vi "Main2_beforerefactoring.vi"() -> ()   [LabVIEW 2021]
uses:
  Hamamatsu_class/SubRegion.ctl
  Application_class/Application.lvclass
  CetoniPump_class/CetoniPump.lvclass
  <vilib>/vision/Image Controls.llb/IMAQ Image.ctl
  Coriolis_Sim_class/Coriolis_Sim.lvclass
  C:/GIT/DensityGradientProject/CoriFlowBFS1Plus_class/CoriFlowBFS1Plus.lvclass
  CoriFlowBFS1Plus_class/CoriFlowBFS1Plus.lvclass
  <vilib>/Utility/error.llb/Error Cluster From Error Code.vi
  <vilib>/ErrorRing/Error Ring.xnode
  AD2_SDK_class/AD2_SDK.lvclass
  Hamamatsu_class/Hamamatsu.lvclass
panel:
  out "Density_g_L":sgl
  out "Temperature(C)":sgl
  out "FLow(ul/min)":sgl
  out "Status":string
  out "Array":T1(array[cluster])
  out "error out":errorcluster
  in  "Tab Control":T2(tab)
  in  "Read Continous":bool
  in  "Go to Level":bool
  in  "Device Configuration Path":string="C:\\Users\\Public\\Documents\\QmixElements\\Projects\\default_project\\Configurations\\double"
  in  "Go to Level":T3
  in  "index":i32
  in  "ReferenceMove":bool
  in  "ReadStatus":bool
  in  "ConfigureSyringe":bool
  in  "SyringeSettings":T4={"index"=0, "SyringeSettings"={"Maximum Piston Stroke (mm)"=100.0, "Inner Diameter (mm)"=12.0}}
  in  "Syringe (only for syringe helper)":T5(ring)=enum."BD 5ml"
  out "Syringe Helper":T6={"Maximum Piston Stroke (mm)"=48.147993421803335, "Inner Diameter (mm)"=12.06}
  in  "Stop ALL Pumps":bool
  in  "CetoniWaitData":T7
  in  "Cetoni Wait for Level":bool
  in  "Center ROI":bool
  in  "Configure ROI":bool
  in  "ROI":T8
  in  "StartLive":bool
  in  "Stop Live":bool
  in  "Open DIO signal helper":bool
  in  "Set Exposure Time":bool
  in  "Read Redout Time":bool
  out "ReadoutTime":dbl
  in  "Exposure (ms)":dbl=5.0 step=1.0
  in  "Start HW Timed Aquisition":bool
  in  "Triggering":T9
  in  "Read Continously?":bool
  in  "Read Coriolis":bool
  in  "Use Coriolis?":bool
  in  "Coriolis VISA resource name":refnum<visa-resource-name>
  in  "Filter(0-1)Min-Max":dbl min=0.0 max=1.0
  out "Display <Replace Me> 2":string
  in  "Exit":bool
  in  "Inject Error<Replace Me>":bool
  in  "Do Something <Replace Me>":bool
  # "DIO0 Pulses at the same time as DIO1,2 and 3 +-offset"
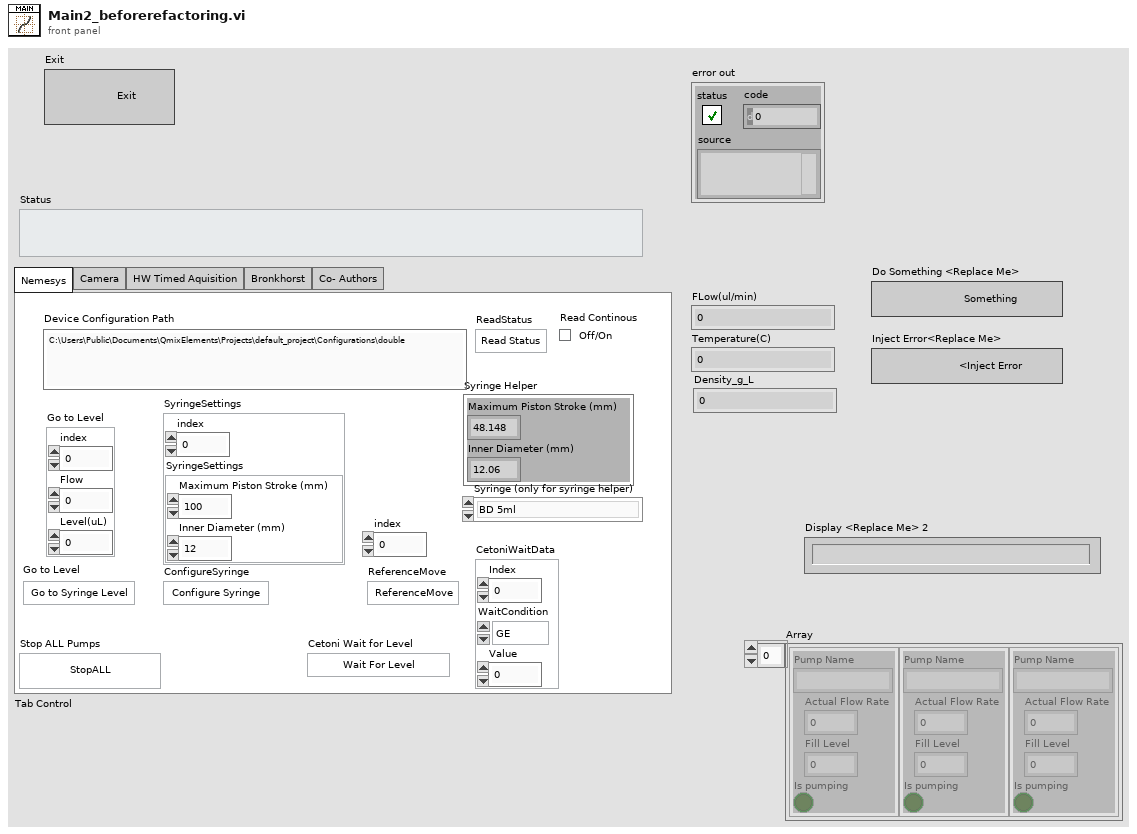
[diagram p1: front panel]
types:
  T1 = cluster{"Pump Name":string, "Actual Flow Rate":dbl, "Fill Level":dbl, "Is pumping":bool}[]
  T2 = enum32{"Nemesys", "Camera", "HW Timed Aquisition", "Bronkhorst", "Co- Authors"}
  T3 = cluster{"index":i32, "Flow":dbl, "Level(uL)":dbl}
  T4 = cluster{"index":i32, "SyringeSettings":cluster{"Maximum Piston Stroke (mm)":dbl, "Inner Diameter (mm)":dbl}}
  T5 = enum16{"BD 1ml", "BD 3ml", "BD 5ml", "BD 10ml", "BD 20ml", "BD 30ml", "BD 50ml", "HSW 1ml"}
  T6 = cluster{"Maximum Piston Stroke (mm)":dbl, "Inner Diameter (mm)":dbl}
  T7 = cluster{"Index":u8, "WaitCondition":enum16{"GE", "LE", "Stopped"}, "Value":dbl}
  T8 = typedef "Hamamatsu.lvclass/SubRegion.ctl" = cluster{"Horizontal Offset":i32, "Vertical Offset":i32, "Horizontal Size":i32, "Vertical Size":i32}
  T9 = cluster{"Pulse Length(ms)":dbl, "DIO0Offset(ms)":dbl, "DIO1 Pulse time (ms)":dbl, "DIO2 Pulse time (ms) 2":dbl, "DIO3 Pulse time (ms) 3":dbl, "EnableDIO3":bool, "EnableDIO2":bool, "EnableDIO1":bool}
  T10 = cluster{"Message":string, "Message Data":variant}
  T11 = cluster{"Fill Level":dbl, "Is pumping":bool, "Actual Flow Rate":dbl}
  T12 = typedef "LVMinMaxIncTypeDef.ctl" = cluster{"Minimum":dbl, "Maximum":dbl, "Increment":dbl}
  T13 = cluster{"H Offset":cluster{"Value":i32, "Limits":T12}, "V Offset":cluster{"Value":i32, "Limits":T12}, "H Size":cluster{"Value":i32, "Limits":T12}, "V Size":cluster{"Value":i32, "Limits":T12}}
  T14 = typedef "Hamamatsu.lvclass/SubRegionLimits.ctl" = cluster{"H Offset":cluster{"Value":i32, "Limits":T12}, "V Offset":cluster{"Value":i32, "Limits":T12}, "H Size":cluster{"Value":i32, "Limits":T12}, "V Size":cluster{"Value":i32, "Limits":T12}}
  T15 = typedef "IMAQ Image.ctl" = refnum<image>
  T16 = enum32{"Invalid", "Standard", "Closed", "Hidden", "Minimized", "Maximized"}
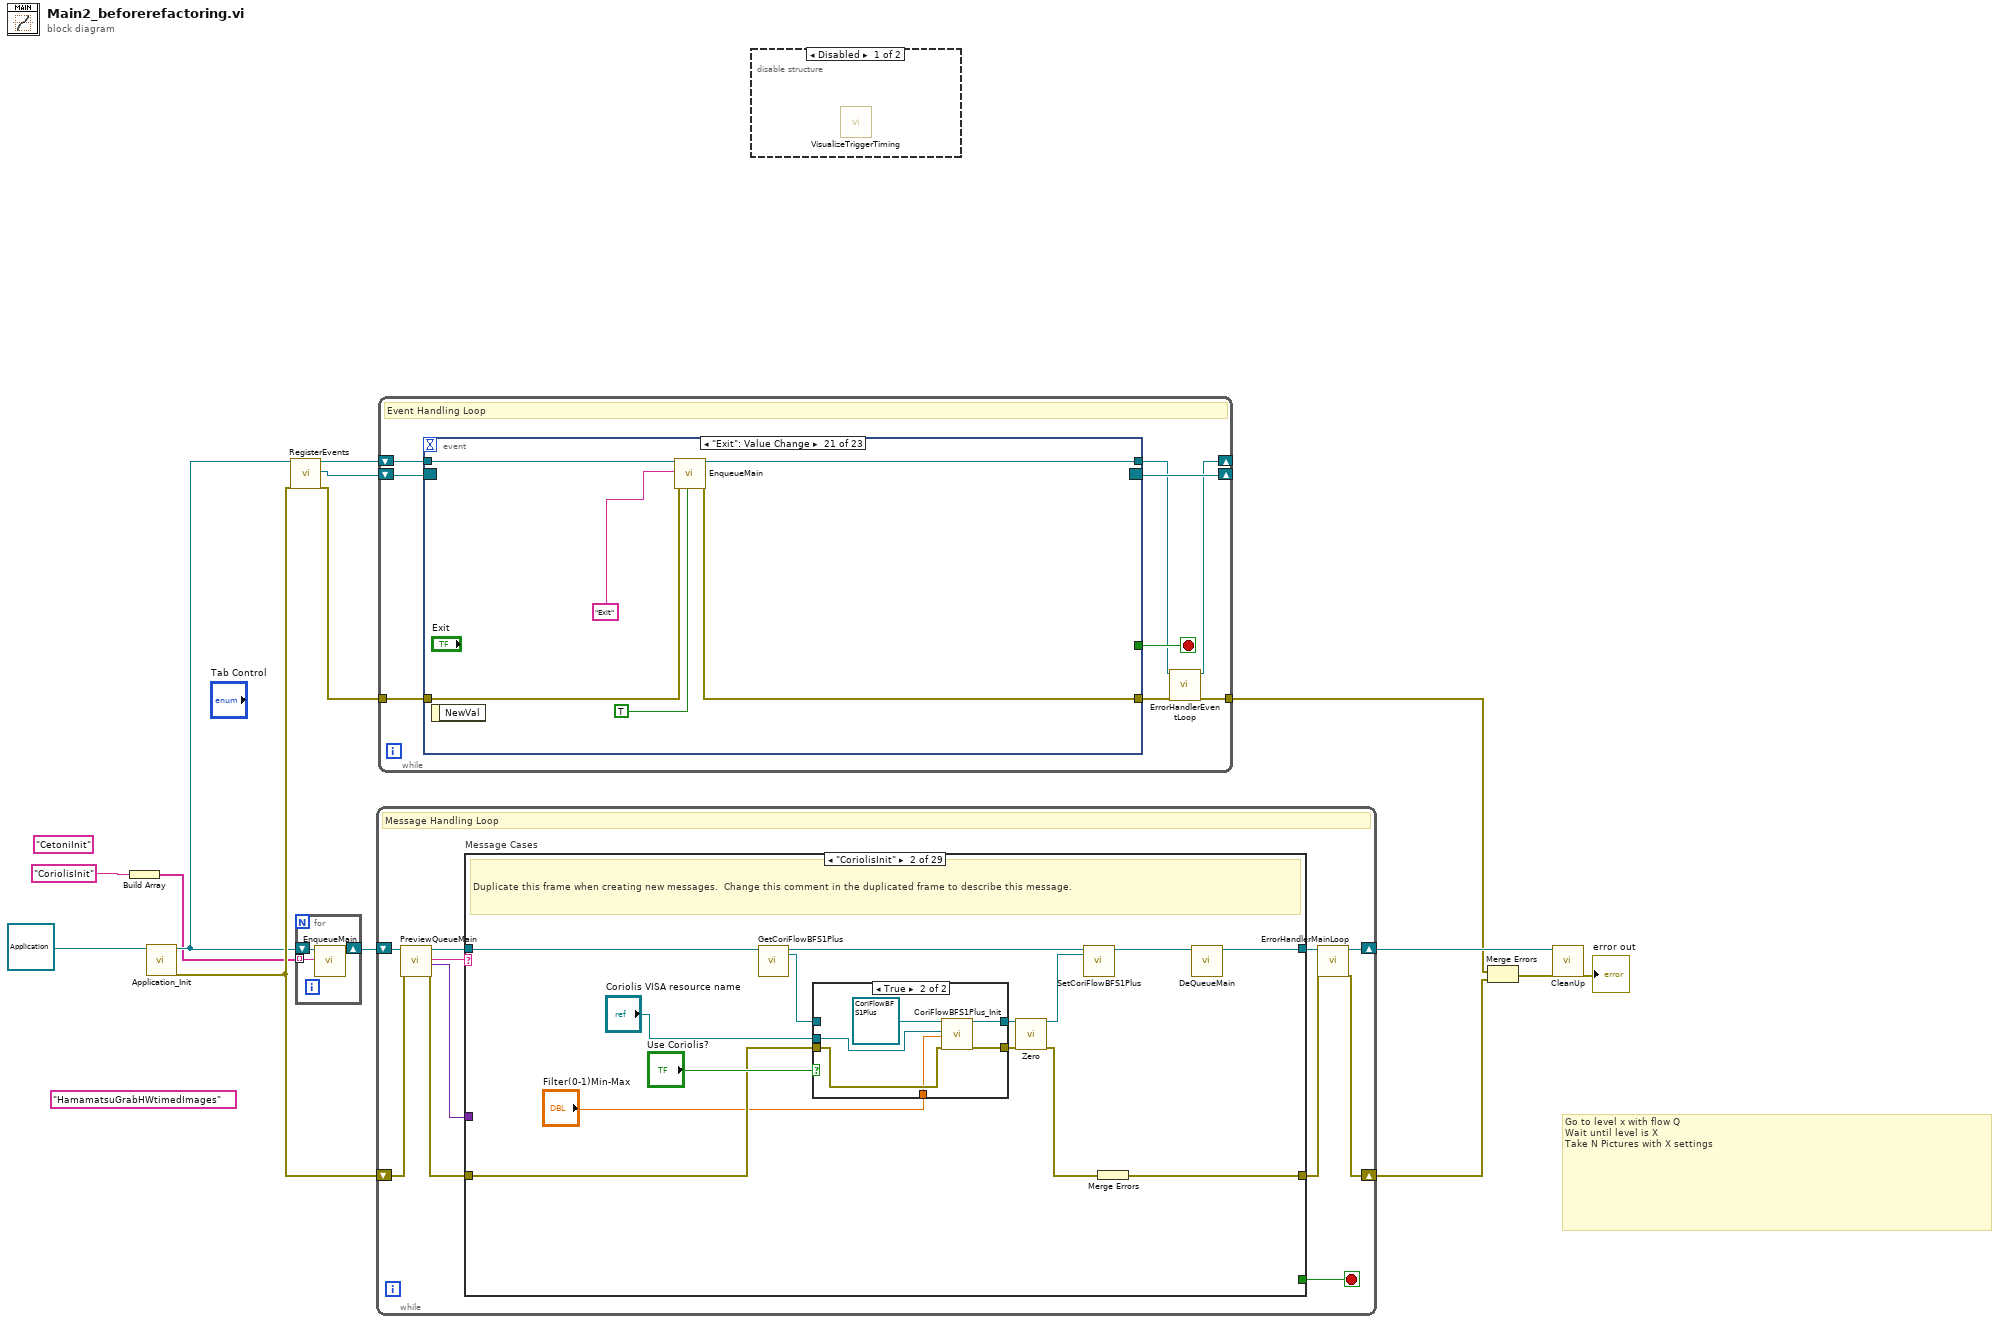
[diagram p0: block diagram]
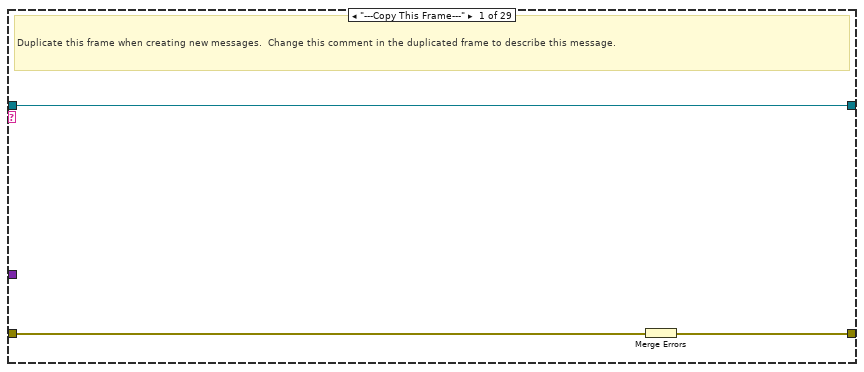
[diagram p3: hidden frame]
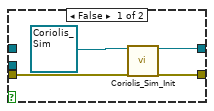
[diagram p4: hidden frame]
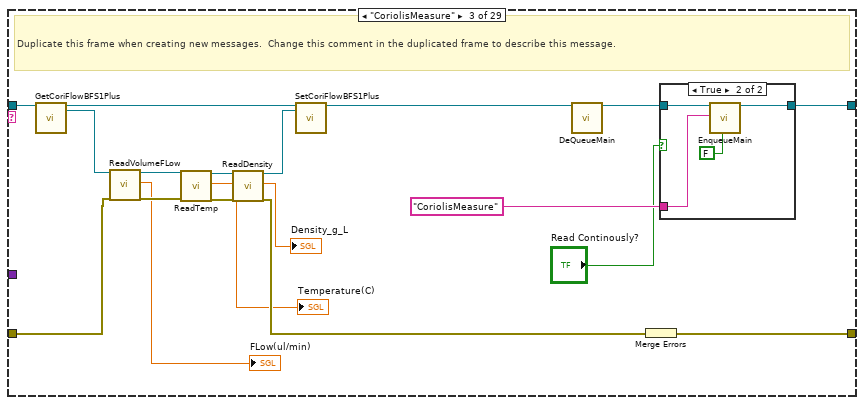
[diagram p5: hidden frame]
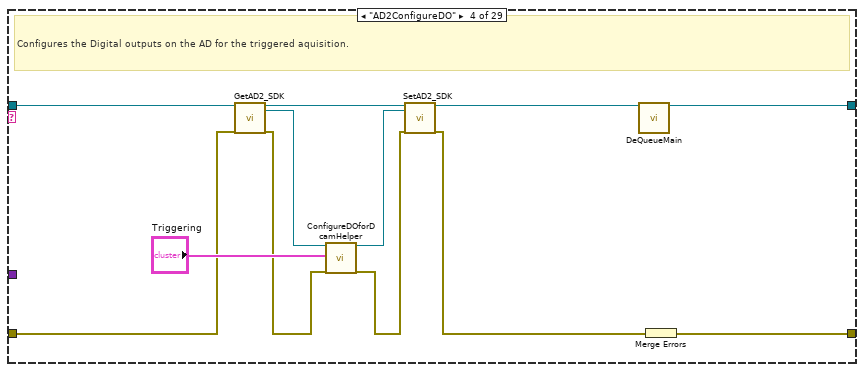
[diagram p7: hidden frame]
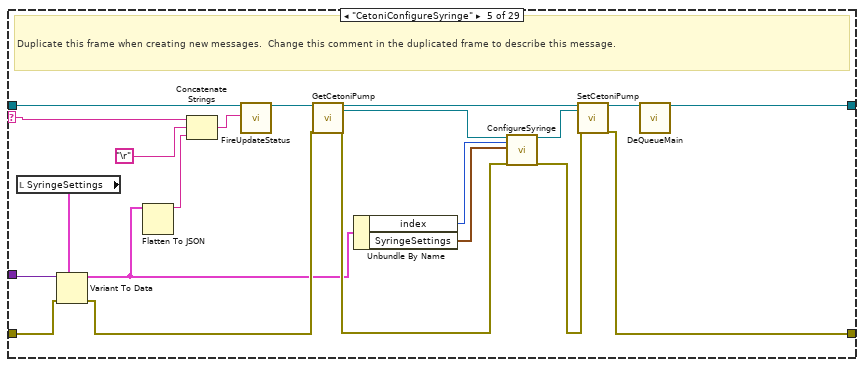
[diagram p8: hidden frame]
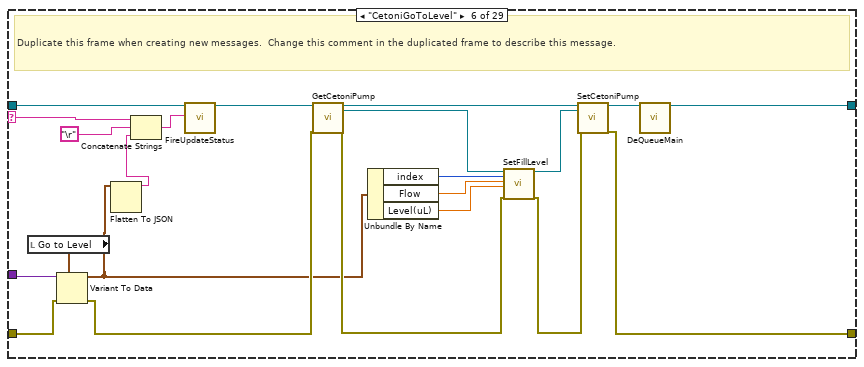
[diagram p9: hidden frame]
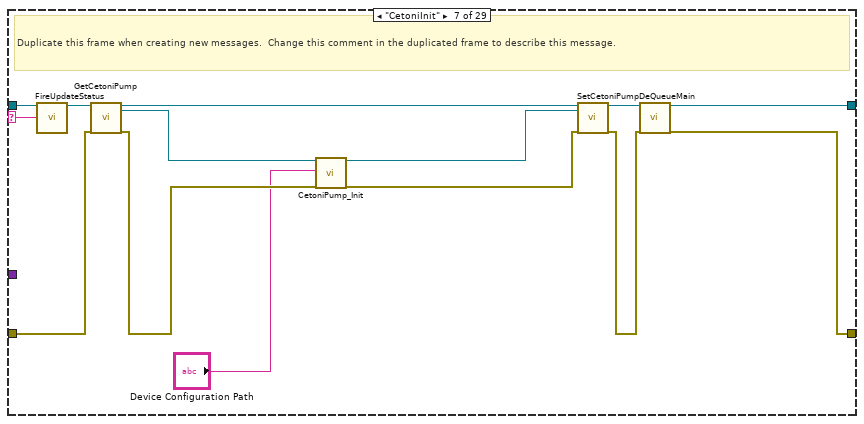
[diagram p10: hidden frame]
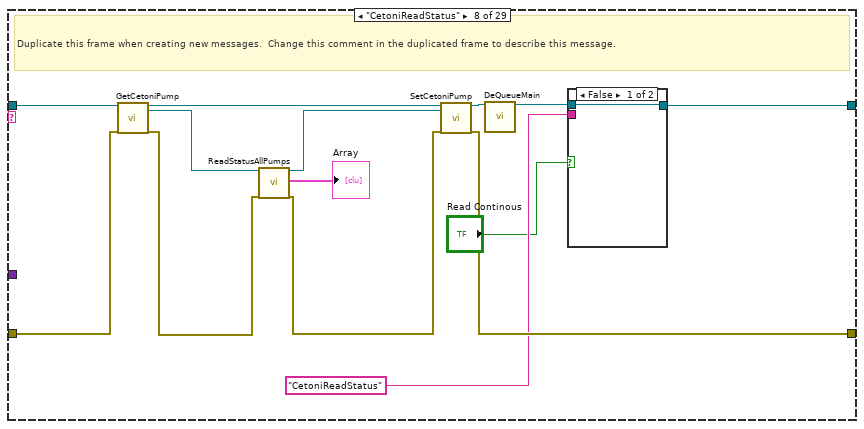
[diagram p11: hidden frame]
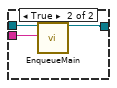
[diagram p12: hidden frame]
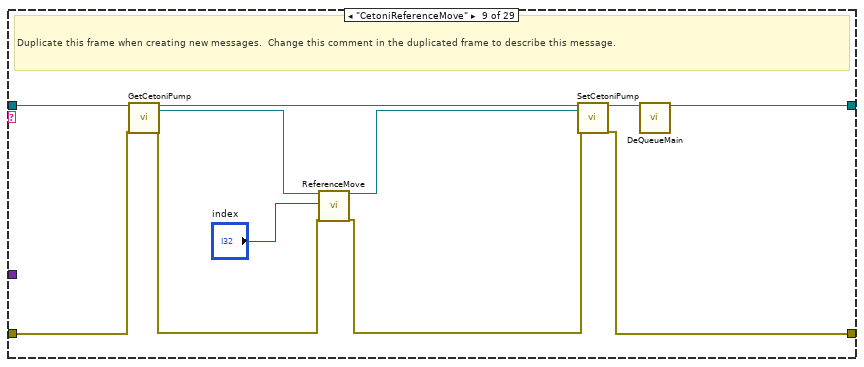
[diagram p13: hidden frame]
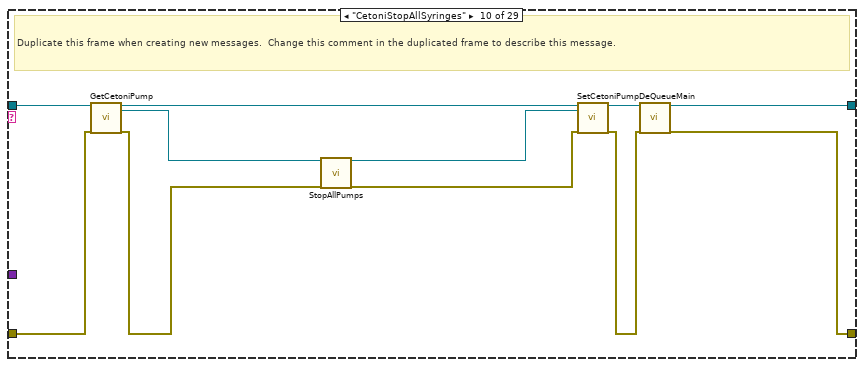
[diagram p14: hidden frame]
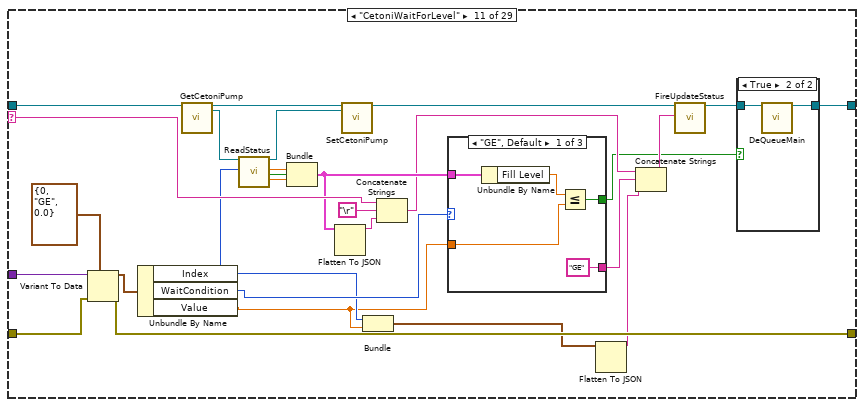
[diagram p15: hidden frame]
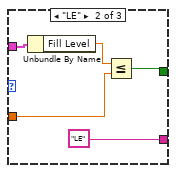
[diagram p17: hidden frame]
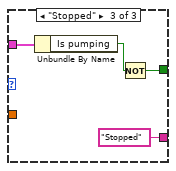
[diagram p18: hidden frame]
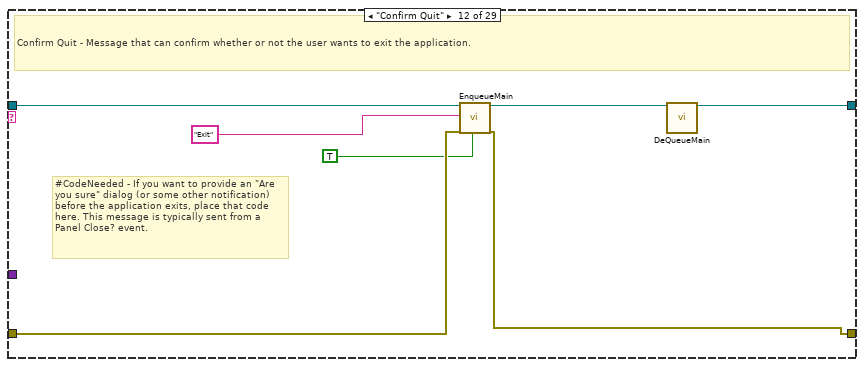
[diagram p19: hidden frame]
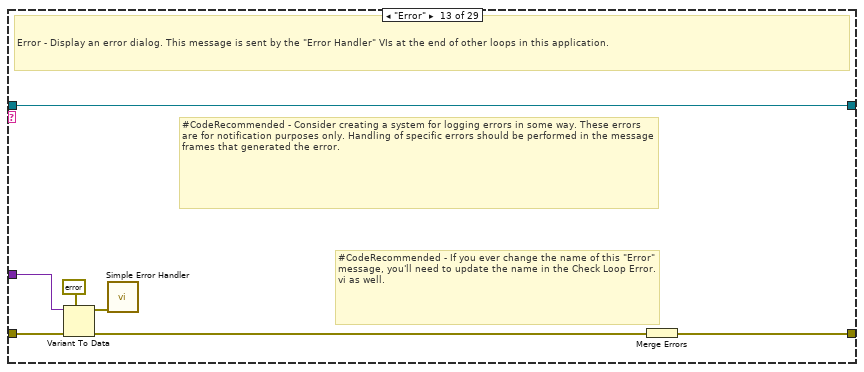
[diagram p20: hidden frame]
diagram:
  (unwired) "HamamatsuGrabHWtimedImages"
  (unwired) "CetoniInit"
  # "Go to level x with flow Q\nWait until level is X\nTake N Pictures with X settings"
  n1 = Build Array("CoriolisInit") -> (w1:string[])
  n2 = call "Application_Init.vi"("object in"=refnum<class "Application.lvclass"> refnum ("Application")) -> ("object out"=w5:refnum<class "Application.lvclass">, "error out"=w10:errorcluster)  [unwired: 17 in]
  n3 = call-dynamic "RegisterEvents.vi"("object in"=w5, "error in (no error)"=w10) -> ("object out"=w12:refnum<class "Application.lvclass">, "Event Registration Refnum"=w13:refnum<event-registration>, "error out"=w11:errorcluster)  [unwired: 15 in]
  n4 = for {
    tunnel: w1 -> [w15] mode=indexing
    shift-right: [w16] -> w3
    shift-left: w5 -> [w17]
    n5 = call-dynamic "EnqueueMain.vi"("object in"=w17, "Message"=w15) -> ("object out"=w16:refnum<class "Application.lvclass">)  [unwired: 16 in, 1 out]
  }
  n6 = while {
    shift-right: [w21] -> w9
    shift-left: w3 -> [w27]
    shift-right: [w22] -> w8
    shift-left: w10 -> [w18]
    stop <- w28 stop-if-true
    # "Message Handling Loop"
    n7 = call-dynamic "PreviewQueueMain.vi"("object in"=w27, "error in (no error)"=w18) -> ("object out"=w26:refnum<class "Application.lvclass">, "Message"=w25:string, "Message Data"=w24:variant, "error out"=w19:errorcluster)  [unwired: 14 in]
    n8 = case "Message Cases" shown="\"CoriolisInit\"" w25 {
      selector: w25 -> [_ _ _ _ w94 w119 w135 _ _ _ w211 _ _ _ _ _ _ _ _ w346 _ _ _ _ _ _ _ _ w449]
      tunnel: w19 -> [w31 w35 w65 w85 w106 w121 w146 w158 w172 w186 w206 w240 w247 w249 w264 w285 w298 w311 w343 w364 w375 w393 w412 w425 w430 w432 w439 w446 _]
      tunnel: [w30 w45 w74 w91 w111 w132 w137 w160 w175 w182 w207 w239 w242 w250 w271 w289 w291 w307 w340 w361 w368 w384 w404 w416 w430 w437 w440 w447 w450] -> w23
      tunnel: [_ _ _ _ _ _ _ _ _ _ _ _ _ TRUE _ _ _ _ _ _ _ _ _ _ _ _ _ _ _] -> w28
      tunnel: w24 -> [_ _ _ _ w108 w115 _ _ _ _ w204 _ w246 _ _ _ _ _ _ _ _ _ _ _ _ w435 _ w445 _]
      tunnel: w26 -> [w29 w44 w73 w87 w92 w133 w147 w161 w176 w187 w216 w236 w241 w251 w270 w288 w301 w313 w345 w347 w378 w399 w415 w428 w429 w436 w438 w441 w448]
      tunnel: [w29 w32 w58 w80 w109 w130 w139 w156 w173 w184 w190 w234 w241 w252 w254 w272 w292 w310 w342 w363 w369 w379 w405 w418 w429 w436 w438 w441 w448] -> w20
      frame "---Copy This Frame---" {
        # "Duplicate this frame when creating new messages.  Change this comment in the duplicated frame to describe this message."
        n9 = Merge Errors(w31) -> (w30:errorcluster)
      }
      frame "CoriolisInit" {
        # "Duplicate this frame when creating new messages.  Change this comment in the duplicated frame to describe this message."
        n10 = call-dynamic "GetCoriFlowBFS1Plus.vi"("object in"=w44) -> ("object out"=w43:refnum<class "Application.lvclass">, "CoriFlowBFS1Plus"=w40:refnum<class "CoriFlowBFS1Plus.lvclass">)  [unwired: 16 in, 1 out]
        n11 = case shown="True" "Use Coriolis?" {
          tunnel: [w49 w55] -> w41
          tunnel: w40 -> [_ _]
          tunnel: w35 -> [w47 w54]
          tunnel: [w46 w53] -> w37
          tunnel: "Coriolis VISA resource name" -> [_ w51]
          tunnel: "Filter(0-1)Min-Max" -> [_ w50]
          frame False {
            n12 = call "Coriolis_Sim_Init.vi"("object in"=refnum<class "Coriolis_Sim.lvclass"> refnum ("Coriolis_Sim"), "error in (no error)"=w47) -> ("object out"=w49:refnum<class "Coriolis_Sim.lvclass">, "error out"=w46:errorcluster)  [unwired: 16 in]
          }
          frame True {
            n13 = call "CoriFlowBFS1Plus_Init.vi"("object in"=refnum<class "CoriFlowBFS1Plus.lvclass"> refnum ("CoriFlowBFS1Plus"), "VISA resource name"=w51, "Filter(0-1)Min-Max"=w50, "error in (no error)"=w54) -> ("object out"=w55:refnum<class "CoriFlowBFS1Plus.lvclass">, "error out"=w53:errorcluster)  [unwired: 14 in]
          }
        }
        n14 = call-dynamic "Zero.vi"("object in"=w41, "error in (no error)"=w37) -> ("object out"=w39:refnum<class "CoriFlowBFS1Plus.lvclass">, "error out"=w36:errorcluster)  [unwired: 16 in]
        n15 = call-dynamic "SetCoriFlowBFS1Plus.vi"("object in"=w43, "CoriFlowBFS1Plus"=w39) -> ("object out"=w42:refnum<class "Application.lvclass">)  [unwired: 16 in, 1 out]
        n16 = Merge Errors(w36) -> (w45:errorcluster)
        n17 = call-dynamic "DeQueueMain.vi"("object in"=w42) -> ("object out"=w32:refnum<class "Application.lvclass">)  [unwired: 15 in, 3 out]
      }
      frame "CoriolisMeasure" {
        # "Duplicate this frame when creating new messages.  Change this comment in the duplicated frame to describe this message."
        n18 = call-dynamic "GetCoriFlowBFS1Plus.vi"("object in"=w73) -> ("object out"=w72:refnum<class "Application.lvclass">, "CoriFlowBFS1Plus"=w66:refnum<class "CoriFlowBFS1Plus.lvclass">)  [unwired: 16 in, 1 out]
        n19 = call-dynamic "ReadVolumeFLow.vi"("object in"=w66, "error in (no error)"=w65) -> ("object out"=w67:refnum<class "CoriFlowBFS1Plus.lvclass">, "FLow(ul/min)"=→"FLow(ul/min)":sgl, "error out"=w64:errorcluster)  [unwired: 15 in]
        n20 = call-dynamic "ReadTemp.vi"("object in"=w67, "error in (no error)"=w64) -> ("object out"=w68:refnum<class "CoriFlowBFS1Plus.lvclass">, "Temperature(C)"=→"Temperature(C)":sgl, "error out"=w63:errorcluster)  [unwired: 15 in]
        n21 = call-dynamic "ReadDensity.vi"("object in"=w68, "error in (no error)"=w63) -> ("object out"=w70:refnum<class "CoriFlowBFS1Plus.lvclass">, "Density_g_L"=→"Density_g_L":sgl, "error out"=w69:errorcluster)  [unwired: 15 in]
        n22 = call-dynamic "SetCoriFlowBFS1Plus.vi"("object in"=w72, "CoriFlowBFS1Plus"=w70) -> ("object out"=w71:refnum<class "Application.lvclass">)  [unwired: 16 in, 1 out]
        n23 = call-dynamic "DeQueueMain.vi"("object in"=w71) -> ("object out"=w59:refnum<class "Application.lvclass">)  [unwired: 15 in, 3 out]
        n24 = Merge Errors(w69) -> (w74:errorcluster)
        n25 = case shown="True" "Read Continously?" {
          tunnel: w59 -> [w75 w79]
          tunnel: [w75 w78] -> w58
          tunnel: "CoriolisMeasure" ("Message") -> [_ w77]
          frame False {
          }
          frame True {
            n26 = call-dynamic "EnqueueMain.vi"("object in"=w79, "Message"=w77, "Priority Message? (F)"=FALSE) -> ("object out"=w78:refnum<class "Application.lvclass">)  [unwired: 15 in, 1 out]
          }
        }
      }
      frame "AD2ConfigureDO" {
        # "Configures the Digital outputs on the AD for the triggered aquisition."
        n27 = call-dynamic "GetAD2_SDK.vi"("object in"=w87, "error in (no error)"=w85) -> ("object out"=w89:refnum<class "Application.lvclass">, "AD2_SDK"=w82:refnum<class "AD2_SDK.lvclass">, "error out"=w86:errorcluster)  [unwired: 15 in]
        n28 = call-dynamic "ConfigureDOforDcamHelper.vi"("object in"=w82, "Pulse Settings"="Triggering", "error in (no error)"=w86) -> ("object out"=w81:refnum<class "AD2_SDK.lvclass">, "error out"=w84:errorcluster)  [unwired: 15 in]
        n29 = call-dynamic "SetAD2_SDK.vi"("object in"=w89, "AD2_SDK"=w81, "error in (no error)"=w84) -> ("object out"=w88:refnum<class "Application.lvclass">, "error out"=w83:errorcluster)  [unwired: 15 in]
        n30 = call-dynamic "DeQueueMain.vi"("object in"=w88) -> ("object out"=w80:refnum<class "Application.lvclass">)  [unwired: 15 in, 3 out]
        n31 = Merge Errors(w83) -> (w91:errorcluster)
      }
      frame "CetoniConfigureSyringe" {
        # "Duplicate this frame when creating new messages.  Change this comment in the duplicated frame to describe this message."
        n32 = local read "SyringeSettings"() -> (w101:T4)
        n33 = Variant To Data(error in=w106, type=w101, Variant=w108) -> (data=w95:T4, error out=w107:errorcluster)
        n34 = Flatten To JSON(anything=w95) -> (JSON string=w96:string)  [unwired: 2 in, 1 out]
        n35 = Concatenate Strings(w94, "\r", w96) -> (w97:string)
        n36 = call-dynamic "FireUpdateStatus.vi"("object in"=w92, "Status"=w97) -> ("object out"=w93:refnum<class "Application.lvclass">)  [unwired: 16 in, 1 out]
        n37 = call-dynamic "GetCetoniPump.vi"("object in"=w93, "error in (no error)"=w107) -> ("object out"=w112:refnum<class "Application.lvclass">, "CetoniPump"=w103:refnum<class "CetoniPump.lvclass">, "error out"=w105:errorcluster)  [unwired: 15 in]
        n38 = Unbundle By Name(w95) -> ("index"=w100:i32, "SyringeSettings"=w99:T6)
        n39 = call-dynamic "ConfigureSyringe.vi"("object in"=w103, "index"=w100, "SyringeSettings"=w99, "error in (no error)"=w105) -> ("object out"=w102:refnum<class "CetoniPump.lvclass">, "error out"=w104:errorcluster)  [unwired: 14 in]
        n40 = call-dynamic "SetCetoniPump.vi"("object in"=w112, "CetoniPump"=w102, "error in (no error)"=w104) -> ("object out"=w110:refnum<class "Application.lvclass">, "error out"=w111:errorcluster)  [unwired: 15 in]
        n41 = call-dynamic "DeQueueMain.vi"("object in"=w110) -> ("object out"=w109:refnum<class "Application.lvclass">)  [unwired: 15 in, 3 out]
      }
      frame "CetoniGoToLevel" {
        # "Duplicate this frame when creating new messages.  Change this comment in the duplicated frame to describe this message."
        n42 = local read "Go to Level"() -> (w120:T3)
        n43 = Variant To Data(error in=w121, type=w120, Variant=w115) -> (data=w114:T3, error out=w122:errorcluster)
        n44 = Flatten To JSON(anything=w114) -> (JSON string=w113:string)  [unwired: 2 in, 1 out]
        n45 = Concatenate Strings(w119, "\r", w113) -> (w116:string)
        n46 = call-dynamic "FireUpdateStatus.vi"("object in"=w133, "Status"=w116) -> ("object out"=w117:refnum<class "Application.lvclass">)  [unwired: 16 in, 1 out]
        n47 = call-dynamic "GetCetoniPump.vi"("object in"=w117, "error in (no error)"=w122) -> ("object out"=w134:refnum<class "Application.lvclass">, "CetoniPump"=w129:refnum<class "CetoniPump.lvclass">, "error out"=w127:errorcluster)  [unwired: 15 in]
        n48 = Unbundle By Name(w114) -> ("index"=w125:i32, "Flow"=w124:dbl, "Level(uL)"=w123:dbl)
        n49 = call-dynamic "SetFillLevel.vi"("object in"=w129, "index"=w125, "Flow"=w124, "Level(ml)"=w123, "error in (no error)"=w127) -> ("object out"=w128:refnum<class "CetoniPump.lvclass">, "error out"=w126:errorcluster)  [unwired: 12 in, 1 out]
        n50 = call-dynamic "SetCetoniPump.vi"("object in"=w134, "CetoniPump"=w128, "error in (no error)"=w126) -> ("object out"=w131:refnum<class "Application.lvclass">, "error out"=w132:errorcluster)  [unwired: 15 in]
        n51 = call-dynamic "DeQueueMain.vi"("object in"=w131) -> ("object out"=w130:refnum<class "Application.lvclass">)  [unwired: 15 in, 3 out]
      }
      frame "CetoniInit" {
        # "Duplicate this frame when creating new messages.  Change this comment in the duplicated frame to describe this message."
        n52 = call-dynamic "FireUpdateStatus.vi"("object in"=w147, "Status"=w135) -> ("object out"=w136:refnum<class "Application.lvclass">)  [unwired: 16 in, 1 out]
        n53 = call-dynamic "GetCetoniPump.vi"("object in"=w136, "error in (no error)"=w146) -> ("object out"=w148:refnum<class "Application.lvclass">, "CetoniPump"=w145:refnum<class "CetoniPump.lvclass">, "error out"=w142:errorcluster)  [unwired: 15 in]
        n54 = call "CetoniPump_Init.vi"("object in"=w145, "Device Configuration Path"="Device Configuration Path", "error in (no error)"=w142) -> ("object out"=w144:refnum<class "CetoniPump.lvclass">, "error out"=w143:errorcluster)  [unwired: 15 in]
        n55 = call-dynamic "SetCetoniPump.vi"("object in"=w148, "CetoniPump"=w144, "error in (no error)"=w143) -> ("object out"=w140:refnum<class "Application.lvclass">, "error out"=w138:errorcluster)  [unwired: 15 in]
        n56 = call-dynamic "DeQueueMain.vi"("object in"=w140, "error in (no error)"=w138) -> ("object out"=w139:refnum<class "Application.lvclass">, "error out"=w137:errorcluster)  [unwired: 14 in, 2 out]
      }
      frame "CetoniReadStatus" {
        # "Duplicate this frame when creating new messages.  Change this comment in the duplicated frame to describe this message."
        n57 = call-dynamic "GetCetoniPump.vi"("object in"=w161, "error in (no error)"=w158) -> ("object out"=w162:refnum<class "Application.lvclass">, "CetoniPump"=w153:refnum<class "CetoniPump.lvclass">, "error out"=w152:errorcluster)  [unwired: 15 in]
        n58 = call-dynamic "ReadStatusAllPumps.vi"("object in"=w153, "error in (no error)"=w152) -> ("object out"=w149:refnum<class "CetoniPump.lvclass">, "Array"=→"Array":T1, "error out"=w151:errorcluster)  [unwired: 15 in]
        n59 = call-dynamic "SetCetoniPump.vi"("object in"=w162, "CetoniPump"=w149, "error in (no error)"=w151) -> ("object out"=w159:refnum<class "Application.lvclass">, "error out"=w160:errorcluster)  [unwired: 15 in]
        n60 = call-dynamic "DeQueueMain.vi"("object in"=w159) -> ("object out"=w157:refnum<class "Application.lvclass">)  [unwired: 15 in, 3 out]
        n61 = case shown="False" "Read Continous" {
          tunnel: w157 -> [w163 w166]
          tunnel: [w163 w165] -> w156
          tunnel: "CetoniReadStatus" ("Message") -> [_ w164]
          frame False {
          }
          frame True {
            n62 = call-dynamic "EnqueueMain.vi"("object in"=w166, "Message"=w164) -> ("object out"=w165:refnum<class "Application.lvclass">)  [unwired: 16 in, 1 out]
          }
        }
      }
      frame "CetoniReferenceMove" {
        # "Duplicate this frame when creating new messages.  Change this comment in the duplicated frame to describe this message."
        n63 = call-dynamic "GetCetoniPump.vi"("object in"=w176, "error in (no error)"=w172) -> ("object out"=w177:refnum<class "Application.lvclass">, "CetoniPump"=w171:refnum<class "CetoniPump.lvclass">, "error out"=w169:errorcluster)  [unwired: 15 in]
        n64 = call-dynamic "ReferenceMove.vi"("object in"=w171, "index"="index", "error in (no error)"=w169) -> ("object out"=w170:refnum<class "CetoniPump.lvclass">, "error out"=w168:errorcluster)  [unwired: 15 in]
        n65 = call-dynamic "SetCetoniPump.vi"("object in"=w177, "CetoniPump"=w170, "error in (no error)"=w168) -> ("object out"=w174:refnum<class "Application.lvclass">, "error out"=w175:errorcluster)  [unwired: 15 in]
        n66 = call-dynamic "DeQueueMain.vi"("object in"=w174) -> ("object out"=w173:refnum<class "Application.lvclass">)  [unwired: 15 in, 3 out]
      }
      frame "CetoniStopAllSyringes" {
        # "Duplicate this frame when creating new messages.  Change this comment in the duplicated frame to describe this message."
        n67 = call-dynamic "GetCetoniPump.vi"("object in"=w187, "error in (no error)"=w186) -> ("object out"=w188:refnum<class "Application.lvclass">, "CetoniPump"=w179:refnum<class "CetoniPump.lvclass">, "error out"=w181:errorcluster)  [unwired: 15 in]
        n68 = call-dynamic "StopAllPumps.vi"("object in"=w179, "error in (no error)"=w181) -> ("object out"=w178:refnum<class "CetoniPump.lvclass">, "error out"=w180:errorcluster)  [unwired: 16 in]
        n69 = call-dynamic "SetCetoniPump.vi"("object in"=w188, "CetoniPump"=w178, "error in (no error)"=w180) -> ("object out"=w185:refnum<class "Application.lvclass">, "error out"=w183:errorcluster)  [unwired: 15 in]
        n70 = call-dynamic "DeQueueMain.vi"("object in"=w185, "error in (no error)"=w183) -> ("object out"=w184:refnum<class "Application.lvclass">, "error out"=w182:errorcluster)  [unwired: 14 in, 2 out]
      }
      frame "CetoniWaitForLevel" {
        n71 = Variant To Data(error in=w206, type=T7 {"Index"=0, "WaitCondition"=enum."GE", "Value"=0.0} ("CetoniWaitData"), Variant=w204) -> (data=w203:T7, error out=w207:errorcluster)
        n72 = Unbundle By Name(w203) -> ("Index"=w194:u8, "WaitCondition"=w202:enum16{"GE", "LE", "Stopped"}, "Value"=w193:dbl)
        n73 = call-dynamic "GetCetoniPump.vi"("object in"=w216) -> ("object out"=w215:refnum<class "Application.lvclass">, "CetoniPump"=w214:refnum<class "CetoniPump.lvclass">)  [unwired: 16 in, 1 out]
        n74 = call-dynamic "ReadStatus.vi"("object in"=w214, "index"=w194) -> ("object out"=w213:refnum<class "CetoniPump.lvclass">, "Fill Level"=w210:dbl, "Is pumping"=w209:bool, "Actual Flow Rate"=w208:dbl)  [unwired: 13 in, 1 out]
        n75 = Bundle("Fill Level"=w210, "Is pumping"=w209, "Actual Flow Rate"=w208) -> (w201:T11)  [unwired: 1 in]
        n76 = Flatten To JSON(anything=w201) -> (JSON string=w198:string)  [unwired: 2 in, 1 out]
        n77 = call-dynamic "SetCetoniPump.vi"("object in"=w215, "CetoniPump"=w213) -> ("object out"=w200:refnum<class "Application.lvclass">)  [unwired: 16 in, 1 out]
        n78 = Bundle("Index"=w194, "Value"=w193) -> (w192:cluster{"Index":u8, "Value":dbl})  [unwired: 1 in]
        n79 = Concatenate Strings(w211, "\r", w198) -> (w197:string)
        n80 = case shown="\"GE\", Default" w202 {
          tunnel: w201 -> [w223 w229 w233]
          tunnel: w193 -> [w222 w227 _]
          tunnel: [w221 w226 w231] -> w189
          tunnel: ["GE" "LE" "Stopped"] -> w196
          frame "GE", Default {
            n81 = Unbundle By Name(w223) -> ("Fill Level"=w224:dbl)
            n82 = Less Or Equal?(x=w224, y=w222) -> (x <= y?=w221:bool)
          }
          frame "LE" {
            n83 = Unbundle By Name(w229) -> ("Fill Level"=w228:dbl)
            n84 = Less Or Equal?(x=w228, y=w227) -> (x <= y?=w226:bool)
          }
          frame "Stopped" {
            n85 = Unbundle By Name(w233) -> ("Is pumping"=w232:bool)
            n86 = Not(x=w232) -> (.not. x?=w231:bool)
          }
        }
        n87 = Flatten To JSON(anything=w192) -> (JSON string=w195:string)  [unwired: 2 in, 1 out]
        n88 = Concatenate Strings(w197, w196, w195) -> (w191:string)
        n89 = call-dynamic "FireUpdateStatus.vi"("object in"=w200, "Status"=w191) -> ("object out"=w199:refnum<class "Application.lvclass">)  [unwired: 16 in, 1 out]
        n90 = case shown="True" w189 {
          tunnel: w199 -> [w217 w219]
          tunnel: [w217 w218] -> w190
          frame False {
          }
          frame True {
            n91 = call-dynamic "DeQueueMain.vi"("object in"=w219) -> ("object out"=w218:refnum<class "Application.lvclass">)  [unwired: 15 in, 3 out]
          }
        }
      }
      frame "Confirm Quit" {
        # "#CodeNeeded - If you want to provide an \"Are you sure\" dialog (or some other notification) before the application exits, place that code here. This message is typically sent from a Panel Close? event."
        # "Confirm Quit - Message that can confirm whether or not the user wants to exit the application."
        n92 = call-dynamic "EnqueueMain.vi"("object in"=w236, "Message"="Exit", "error in (no error)"=w240, "Priority Message? (F)"=TRUE) -> ("object out"=w237:refnum<class "Application.lvclass">, "error out"=w239:errorcluster)  [unwired: 14 in]
        n93 = call-dynamic "DeQueueMain.vi"("object in"=w237) -> ("object out"=w234:refnum<class "Application.lvclass">)  [unwired: 15 in, 3 out]
      }
      frame "Error" {
        # "#CodeRecommended - If you ever change the name of this \"Error\" message, you'll need to update the name in the Check Loop Error.vi as well."
        # "#CodeRecommended - Consider creating a system for logging errors in some way. These errors are for notification purposes only. Handling of specific errors should be performed in the message frames that generated the error."
        # "Error - Display an error dialog. This message is sent by the \"Error Handler\" VIs at the end of other loops in this application."
        n94 = Variant To Data(error in=w247, type=errorcluster {"status"=FALSE, "code"=0, "source"=""} ("error constant"), Variant=w246) -> (data=w244:errorcluster, error out=w243:errorcluster)
        n95 = call <vilib>:"Simple Error Handler.vi"("error in (no error)"=w244) -> ()  [unwired: 4 in, 5 out]
        n96 = Merge Errors(w243) -> (w242:errorcluster)
      }
      frame "Exit" {
        # "Stop the VI"
        # "Release the message queue reference"
        # "#CodeNeeded - Add any required cleanup code here. Note that if 'Exit' was called as a result of an error, an error dialog will be displayed. Add any custom error handling for an 'Exit' condition here as well."
        # "Exit - Exit the application."
        n97 = call <vilib>:"Simple Error Handler.vi"("error in (no error)"=w249) -> ("error out"=w248:errorcluster)  [unwired: 4 in, 4 out]
        n98 = call-dynamic "FireStopEvent.vi"("object in"=w251, "error in (no error)"=w248) -> ("object out"=w252:refnum<class "Application.lvclass">, "error out"=w250:errorcluster)  [unwired: 16 in]
      }
      frame "HamamatsuCenterROI" {
        # "Duplicate this frame when creating new messages.  Change this comment in the duplicated frame to describe this message."
        n99 = call-dynamic "GetHamamatsu.vi"("object in"=w270, "error in (no error)"=w264) -> ("object out"=w269:refnum<class "Application.lvclass">, "Hamamatsu"=w267:refnum<class "Hamamatsu.lvclass">, "error out"=w265:errorcluster)  [unwired: 15 in]
        n100 = call-dynamic "CenterROI.vi"("object in"=w267, "error in (no error)"=w265) -> ("object out"=w266:refnum<class "Hamamatsu.lvclass">, "Sub Region"=w259:T13, "error out"=w263:errorcluster)  [unwired: 15 in]
        n101 = call-dynamic "SetHamamatsu.vi"("object in"=w269, "Hamamatsu"=w266, "error in (no error)"=w263) -> ("object out"=w268:refnum<class "Application.lvclass">, "error out"=w262:errorcluster)  [unwired: 15 in]
        n102 = Unbundle By Name(w259) -> ("H Offset.Value"=w258:i32, "V Offset.Value"=w257:i32, "H Size.Value"=w256:i32, "V Size.Value"=w255:i32)
        n103 = Bundle By Name(cluster=T8 {"Horizontal Offset"=0, "Vertical Offset"=0, "Horizontal Size"=0, "Vertical Size"=0} ("Sub Region"), "Horizontal Offset"=w258, "Vertical Offset"=w257, "Horizontal Size"=w256, "Vertical Size"=w255) -> (w260:T8)
        n104 = call-dynamic "DeQueueMain.vi"("object in"=w268) -> ("object out"=w254:refnum<class "Application.lvclass">)  [unwired: 15 in, 3 out]
        n105 = local write "ROI"(w260) -> ()
        n106 = Merge Errors(w262) -> (w271:errorcluster)
      }
      frame "HamamatsuConfigureROI" {
        # "Duplicate this frame when creating new messages.  Change this comment in the duplicated frame to describe this message."
        n107 = call-dynamic "GetHamamatsu.vi"("object in"=w288, "error in (no error)"=w285) -> ("object out"=w287:refnum<class "Application.lvclass">, "Hamamatsu"=w283:refnum<class "Hamamatsu.lvclass">, "error out"=w281:errorcluster)  [unwired: 15 in]
        n108 = call-dynamic "ConfigureROI.vi"("object in"=w283, "Sub Region"="ROI", "error in (no error)"=w281) -> ("object out"=w282:refnum<class "Hamamatsu.lvclass">, "SubRegionLimits"=w279:T14, "error out"=w280:errorcluster)  [unwired: 14 in]
        n109 = call-dynamic "SetHamamatsu.vi"("object in"=w287, "Hamamatsu"=w282, "error in (no error)"=w280) -> ("object out"=w286:refnum<class "Application.lvclass">, "error out"=w284:errorcluster)  [unwired: 15 in]
        n110 = Unbundle By Name(w279) -> ("H Offset.Value"=w276:i32, "V Offset.Value"=w275:i32, "H Size.Value"=w274:i32, "V Size.Value"=w273:i32)
        n111 = Merge Errors(w284) -> (w289:errorcluster)
        n112 = Bundle By Name(cluster="ROI", "Horizontal Offset"=w276, "Vertical Offset"=w275, "Horizontal Size"=w274, "Vertical Size"=w273) -> (w277:T8)
        n113 = call-dynamic "DeQueueMain.vi"("object in"=w286) -> ("object out"=w272:refnum<class "Application.lvclass">)  [unwired: 15 in, 3 out]
        n114 = local write "ROI"(w277) -> ()
      }
      frame "HamamatsuGetReadoutTime" {
        # "Duplicate this frame when creating new messages.  Change this comment in the duplicated frame to describe this message."
        n115 = call-dynamic "GetHamamatsu.vi"("object in"=w301, "error in (no error)"=w298) -> ("object out"=w300:refnum<class "Application.lvclass">, "Hamamatsu"=w296:refnum<class "Hamamatsu.lvclass">, "error out"=w294:errorcluster)  [unwired: 15 in]
        n116 = call-dynamic "ReadReadoutTime.vi"("object in"=w296, "error in (no error)"=w294) -> ("object out"=w295:refnum<class "Hamamatsu.lvclass">, "ReadoutTime"=→"ReadoutTime":dbl, "error out"=w293:errorcluster)  [unwired: 15 in]
        n117 = call-dynamic "SetHamamatsu.vi"("object in"=w300, "Hamamatsu"=w295, "error in (no error)"=w293) -> ("object out"=w299:refnum<class "Application.lvclass">, "error out"=w297:errorcluster)  [unwired: 15 in]
        n118 = call-dynamic "DeQueueMain.vi"("object in"=w299, "error in (no error)"=w297) -> ("object out"=w292:refnum<class "Application.lvclass">, "error out"=w291:errorcluster)  [unwired: 14 in, 2 out]
      }
      frame "HamamatsuGrabHWtimedImages" {
        # "Duplicate this frame when creating new messages.  Change this comment in the duplicated frame to describe this message."
        n119 = call-dynamic "GetHamamatsu.vi"("object in"=w313, "error in (no error)"=w311) -> ("object out"=w312:refnum<class "Application.lvclass">, "Hamamatsu"=w309:refnum<class "Hamamatsu.lvclass">, "error out"=w308:errorcluster)  [unwired: 15 in]
        n120 = call-dynamic "CaptureHWSynced.vi"("object in"=w309, "error in (no error)"=w308) -> ("object out"=w306:refnum<class "Hamamatsu.lvclass">, "AllFramesAvailable?"=w302:bool, "error out"=w304:errorcluster)  [unwired: 13 in, 2 out]
        n121 = call-dynamic "SetHamamatsu.vi"("object in"=w312, "Hamamatsu"=w306, "error in (no error)"=w304) -> ("object out"=w305:refnum<class "Application.lvclass">, "error out"=w303:errorcluster)  [unwired: 15 in]
        n122 = case shown="True" w302 {
          tunnel: [w315 w319] -> w307
          tunnel: w303 -> [w315 w327]
          tunnel: w306 -> [_ w326]
          tunnel: w305 -> [w314 w325]
          tunnel: [w314 w322] -> w310
          frame False {
          }
          frame True {
            (unwired) variant ("Message Data")
            n123 = call-dynamic "GetImages.vi"("object in"=w326, "error in (no error)"=w327) -> ("HWSyncedImages"=w316:T15[], "error out"=w324:errorcluster)  [unwired: 15 in, 1 out]
            n124 = call-dynamic "DeQueueMain.vi"("object in"=w325, "error in (no error)"=w324) -> ("object out"=w323:refnum<class "Application.lvclass">, "error out"=w320:errorcluster)  [unwired: 14 in, 2 out]
            n125 = Bundle By Name(cluster=T10 {"Message"="", "Message Data"=variant} ("event data"), "Message"="UpdateHWTimed", "Message Data"=w316) -> (w317:T10)
            n126 = call-dynamic "FireMessageEvent.vi"("object in"=w323, "event data"=w317, "error in (no error)"=w320) -> ("object out"=w322:refnum<class "Application.lvclass">, "error out"=w319:errorcluster)  [unwired: 15 in]
          }
        }
      }
      frame "HamamatsuGrabLive" {
        # "Duplicate this frame when creating new messages.  Change this comment in the duplicated frame to describe this message."
        n127 = call-dynamic "GetHamamatsu.vi"("object in"=w345, "error in (no error)"=w343) -> ("object out"=w344:refnum<class "Application.lvclass">, "Hamamatsu"=w339:refnum<class "Hamamatsu.lvclass">, "error out"=w337:errorcluster)  [unwired: 15 in]
        n128 = call-dynamic "CaptureSnapshot.vi"("object in"=w339, "error in (no error)"=w337) -> ("object out"=w338:refnum<class "Hamamatsu.lvclass">, "FreeRunningImage"=w328:T15, "error out"=w336:errorcluster)  [unwired: 14 in, 1 out]
        n129 = call-dynamic "SetHamamatsu.vi"("object in"=w344, "Hamamatsu"=w338, "error in (no error)"=w336) -> ("object out"=w333:refnum<class "Application.lvclass">, "error out"=w341:errorcluster)  [unwired: 15 in]
        n130 = Bundle By Name(cluster=T10 {"Message"="", "Message Data"=variant} ("event data"), "Message"="UpdateLive", "Message Data"=w328) -> (w330:T10)
        n131 = call-dynamic "FireMessageEvent.vi"("object in"=w333, "event data"=w330) -> ("object out"=w329:refnum<class "Application.lvclass">)  [unwired: 16 in, 1 out]
        n132 = call-dynamic "DeQueueMain.vi"("object in"=w329) -> ("object out"=w334:refnum<class "Application.lvclass">)  [unwired: 15 in, 3 out]
        n133 = call-dynamic "EnqueueMain.vi"("object in"=w334, "Message"="HamamatsuGrabLive", "error in (no error)"=w341) -> ("object out"=w342:refnum<class "Application.lvclass">, "error out"=w340:errorcluster)  [unwired: 15 in]
      }
      frame "HamamatsuInit" {
        # "Duplicate this frame when creating new messages.  Change this comment in the duplicated frame to describe this message."
        n134 = call-dynamic "FireUpdateStatus.vi"("object in"=w347, "Status"=w346) -> ("object out"=w348:refnum<class "Application.lvclass">)  [unwired: 16 in, 1 out]
        n135 = call-dynamic "GetHamamatsu.vi"("object in"=w348, "error in (no error)"=w364) -> ("object out"=w366:refnum<class "Application.lvclass">, "Hamamatsu"=w360:refnum<class "Hamamatsu.lvclass">, "error out"=w359:errorcluster)  [unwired: 15 in]
        n136 = call "Hamamatsu_Init.vi"("object in"=w360, "error in (no error)"=w359) -> ("object out"=w358:refnum<class "Hamamatsu.lvclass">, "error out"=w357:errorcluster)  [unwired: 16 in]
        n137 = call-dynamic "OpenCamera.vi"("object in"=w358, "error in (no error)"=w357) -> ("object out"=w354:refnum<class "Hamamatsu.lvclass">, "error out"=w352:errorcluster)  [unwired: 14 in, 2 out]
        n138 = control-ref of="ROI"() -> (w356:refnum<vi>)
        n139 = call-dynamic "ReadSubregionLimitsandValue.vi"("object in"=w354, "error in (no error)"=w352) -> ("object out"=w353:refnum<class "Hamamatsu.lvclass">, "Sub Region"=w350:T13, "error out"=w351:errorcluster)  [unwired: 15 in]
        n140 = call-dynamic "UpdateRoiLimits.vi"("object in"=w353, "reference to front panel item"=w356, "SubRegionLimits"=w350, "error in (no error)"=w351) -> ("object out"=w355:refnum<class "Hamamatsu.lvclass">, "error out"=w349:errorcluster)  [unwired: 14 in]
        n141 = call-dynamic "SetHamamatsu.vi"("object in"=w366, "Hamamatsu"=w355, "error in (no error)"=w349) -> ("object out"=w365:refnum<class "Application.lvclass">, "error out"=w362:errorcluster)  [unwired: 15 in]
        n142 = call-dynamic "DeQueueMain.vi"("object in"=w365, "error in (no error)"=w362) -> ("object out"=w363:refnum<class "Application.lvclass">, "error out"=w361:errorcluster)  [unwired: 14 in, 2 out]
      }
      frame "HamamatsuSetExposureTime" {
        # "Duplicate this frame when creating new messages.  Change this comment in the duplicated frame to describe this message."
        n143 = call-dynamic "GetHamamatsu.vi"("object in"=w378, "error in (no error)"=w375) -> ("object out"=w377:refnum<class "Application.lvclass">, "Hamamatsu"=w373:refnum<class "Hamamatsu.lvclass">, "error out"=w371:errorcluster)  [unwired: 15 in]
        n144 = call-dynamic "ConfigureExposureTime.vi"("object in"=w373, "ExposureTime(ms)"="Exposure (ms)", "error in (no error)"=w371) -> ("object out"=w372:refnum<class "Hamamatsu.lvclass">, "error out"=w370:errorcluster)  [unwired: 15 in]
        n145 = call-dynamic "SetHamamatsu.vi"("object in"=w377, "Hamamatsu"=w372, "error in (no error)"=w370) -> ("object out"=w376:refnum<class "Application.lvclass">, "error out"=w374:errorcluster)  [unwired: 15 in]
        n146 = call-dynamic "DeQueueMain.vi"("object in"=w376, "error in (no error)"=w374) -> ("object out"=w369:refnum<class "Application.lvclass">, "error out"=w368:errorcluster)  [unwired: 14 in, 2 out]
      }
      frame "HamamatsuStartHWTimedAquisition" {
        n147 = call-dynamic "GetHamamatsu.vi"("object in"=w399, "error in (no error)"=w393) -> ("object out"=w398:refnum<class "Application.lvclass">, "Hamamatsu"=w396:refnum<class "Hamamatsu.lvclass">, "error out"=w394:errorcluster)  [unwired: 15 in]
        n148 = call-dynamic "ConfigureHWSynced.vi"("object in"=w396, "FramesPerAquisionCycle"=2, "CameraBufferSize"=3, "error in (no error)"=w394) -> ("object out"=w383:refnum<class "Hamamatsu.lvclass">, "error out"=w381:errorcluster)  [unwired: 14 in]
        n149 = call-dynamic "StartCapture.vi"("object in"=w383, "error in (no error)"=w381) -> ("object out"=w382:refnum<class "Hamamatsu.lvclass">, "error out"=w380:errorcluster)  [unwired: 16 in]
        n150 = call-dynamic "SetHamamatsu.vi"("object in"=w398, "Hamamatsu"=w382, "error in (no error)"=w380) -> ("object out"=w392:refnum<class "Application.lvclass">, "error out"=w387:errorcluster)  [unwired: 15 in]
        n151 = call-dynamic "GetAD2_SDK.vi"("object in"=w392, "error in (no error)"=w387) -> ("object out"=w391:refnum<class "Application.lvclass">, "AD2_SDK"=w389:refnum<class "AD2_SDK.lvclass">, "error out"=w386:errorcluster)  [unwired: 15 in]
        n152 = call-dynamic "PCTrig.vi"("object in"=w389, "error in (no error)"=w386) -> ("object out"=w388:refnum<class "AD2_SDK.lvclass">, "error out"=w385:errorcluster)  [unwired: 16 in]
        n153 = call-dynamic "SetAD2_SDK.vi"("object in"=w391, "AD2_SDK"=w388, "error in (no error)"=w385) -> ("object out"=w390:refnum<class "Application.lvclass">, "error out"=w384:errorcluster)  [unwired: 15 in]
        n154 = call-dynamic "DeQueueMain.vi"("object in"=w390) -> ("object out"=w379:refnum<class "Application.lvclass">)  [unwired: 15 in, 3 out]
      }
      frame "HamamatsuStartLive" {
        # "Duplicate this frame when creating new messages.  Change this comment in the duplicated frame to describe this message."
        n155 = call-dynamic "GetHamamatsu.vi"("object in"=w415, "error in (no error)"=w412) -> ("object out"=w414:refnum<class "Application.lvclass">, "Hamamatsu"=w411:refnum<class "Hamamatsu.lvclass">, "error out"=w410:errorcluster)  [unwired: 15 in]
        n156 = call-dynamic "ConfigureSnapshot.vi"("object in"=w411, "error in (no error)"=w410) -> ("object out"=w409:refnum<class "Hamamatsu.lvclass">, "error out"=w407:errorcluster)  [unwired: 16 in]
        n157 = call-dynamic "StartCapture.vi"("object in"=w409, "error in (no error)"=w407) -> ("object out"=w408:refnum<class "Hamamatsu.lvclass">, "error out"=w406:errorcluster)  [unwired: 16 in]
        n158 = call-dynamic "SetHamamatsu.vi"("object in"=w414, "Hamamatsu"=w408, "error in (no error)"=w406) -> ("object out"=w413:refnum<class "Application.lvclass">, "error out"=w402:errorcluster)  [unwired: 15 in]
        n159 = call-dynamic "DeQueueMain.vi"("object in"=w413, "error in (no error)"=w402) -> ("object out"=w403:refnum<class "Application.lvclass">, "error out"=w401:errorcluster)  [unwired: 14 in, 2 out]
        n160 = call-dynamic "EnqueueMain.vi"("object in"=w403, "Message"="HamamatsuGrabLive", "error in (no error)"=w401) -> ("object out"=w405:refnum<class "Application.lvclass">, "error out"=w404:errorcluster)  [unwired: 15 in]
      }
      frame "HamamatsuStopLive" {
        # "Duplicate this frame when creating new messages.  Change this comment in the duplicated frame to describe this message."
        n161 = call-dynamic "GetHamamatsu.vi"("object in"=w428, "error in (no error)"=w425) -> ("object out"=w427:refnum<class "Application.lvclass">, "Hamamatsu"=w423:refnum<class "Hamamatsu.lvclass">, "error out"=w421:errorcluster)  [unwired: 15 in]
        n162 = call-dynamic "StopCapture.vi"("object in"=w423, "error in (no error)"=w421) -> ("object out"=w422:refnum<class "Hamamatsu.lvclass">, "error out"=w420:errorcluster)  [unwired: 16 in]
        n163 = call-dynamic "SetHamamatsu.vi"("object in"=w427, "Hamamatsu"=w422, "error in (no error)"=w420) -> ("object out"=w426:refnum<class "Application.lvclass">, "error out"=w424:errorcluster)  [unwired: 15 in]
        n164 = call-dynamic "DeQueueMain.vi"("object in"=w426, "error in (no error)"=w424) -> ("object out"=w419:refnum<class "Application.lvclass">, "error out"=w417:errorcluster)  [unwired: 14 in, 2 out]
        n165 = call-dynamic "FlushQueueMain.vi"("object in"=w419, "error in (no error)"=w417) -> ("object out"=w418:refnum<class "Application.lvclass">, "error out"=w416:errorcluster)  [unwired: 15 in, 1 out]
      }
      frame "Initialize" {
        # "Initialize - All initialization work should take place in this message, since other loops can potentially enqueue messages that execute immediately after this one."
      }
      frame "InjectError" {
        # "Something Else - Replace this message with functionality for your own application."
        n166 = Variant To Data(error in=w432, type=errorcluster {"status"=FALSE, "code"=0, "source"=""} ("error in (no error)"), Variant=w435) -> (data=w431:errorcluster, error out=w433:errorcluster)
        n167 = Merge Errors(w431, w433) -> (w437:errorcluster)
      }
      frame "Something" {
        # "Send string to \"Update Display\" message"
        # "#CodeNeeded - Perform whatever actions correspond to the \"Something\" message."
        # "Something - Replace this message with functionality for your own application."
        n168 = Merge Errors(w439) -> (w440:errorcluster)
      }
      frame "Update Display" {
        # "#CodeRecommended - If you wish to decouple the Message Handling Loop from your user interface, consider creating User Events (like the \"Stop\" event in this VI) to message the Event Handling Loop whenever the user interface needs updating."
        # "Update Display - Convert the message data to a string to display in the Data Display indicator."
        n169 = Variant To Data(error in=w446, type="", Variant=w445) -> (data=→"Display <Replace Me> 2":string, error out=w443:errorcluster)
        n170 = Merge Errors(w443) -> (w447:errorcluster)
      }
      frame Default {
        # "'Default' case only runs if there is a message that isn't defined in any of the other cases.  Output a programming error."
        n171 = xnode "Error Ring"("parameter 0"=w449) -> ("error out"=w450:errorcluster)
      }
    }
    n172 = call-dynamic "ErrorHandlerMainLoop.vi"("object in"=w20, "error in (no error)"=w23) -> ("object out"=w21:refnum<class "Application.lvclass">, "error out"=w22:errorcluster)  [unwired: 16 in]
  }
  n173 = while {
    shift-right: [w465] -> _
    shift-left: w13 -> [w466]
    tunnel: [w460] -> w7
    shift-right: [w458] -> _
    shift-left: w12 -> [w463]
    tunnel: w11 -> [w462]
    stop <- w464 stop-if-true
    # "Event Handling Loop"
    n174 = event shown="[20] \"Exit\": Value Change" {
      selector: w466 -> [_ _ _ _ _ _ _ _ _ _ _ _ _ _ _ _ _ _ _ _ _ _ _]
      dyn-events: [_ _ _ _ _ _ _ _ _ _ _ _ _ _ _ _ _ _ _ _ _ _ _] -> w465
      timeout: _ -> [_ _ _ _ _ _ _ _ _ _ _ _ _ _ _ _ _ _ _ _ _ _ _]
      tunnel: [_ _ _ _ _ _ _ _ _ _ _ _ _ _ _ _ _ _ _ _ _ TRUE ("Discard?") _] -> w464
      tunnel: [w468 w473 w479 w483 w488 w493 w498 w503 w508 w513 w532 w535 w540 w546 w551 _ w561 w567 w573 w578 w580 _ w589] -> w461
      tunnel: w463 -> [w471 w476 w482 w486 w491 w496 w501 w506 w511 w516 w533 w538 w543 w549 w554 w558 w564 w570 w572 w579 w585 w586 w592]
      tunnel: [w470 w475 w481 w485 w490 w495 w500 w505 w510 w515 w533 w537 w542 w548 w553 w558 w563 w569 w571 w579 w584 w586 w592] -> w459
      tunnel: w462 -> [w467 w472 w478 w483 w487 w492 w497 w502 w507 w512 w532 w534 w539 w545 w550 _ w560 w566 w574 w578 w581 _ w590]
      event "Do Something <Replace Me>": Value Change {
        n175 = event-data() -> ()  [unwired: 1 in, 1 out]
        n176 = call-dynamic "EnqueueMain.vi"("object in"=w471, "Message"="Something", "error in (no error)"=w467) -> ("object out"=w470:refnum<class "Application.lvclass">, "error out"=w468:errorcluster)  [unwired: 15 in]
      }
      event "Start HW Timed Aquisition": Value Change {
        n177 = event-data() -> ()  [unwired: 1 in, 1 out]
        n178 = call-dynamic "EnqueueMain.vi"("object in"=w476, "Message"="HamamatsuStartHWTimedAquisition", "error in (no error)"=w472) -> ("object out"=w475:refnum<class "Application.lvclass">, "error out"=w473:errorcluster)  [unwired: 15 in]
      }
      event "Cetoni Wait for Level": Value Change {
        n179 = event-data() -> ()  [unwired: 1 in, 1 out]
        n180 = call-dynamic "EnqueueMain.vi"("object in"=w482, "Message"="CetoniWaitForLevel", "Message Data"="CetoniWaitData", "error in (no error)"=w478) -> ("object out"=w481:refnum<class "Application.lvclass">, "error out"=w479:errorcluster)  [unwired: 14 in]
      }
      event "Read Coriolis": Value Change {
        n181 = event-data() -> ()  [unwired: 1 in, 2 out]
        n182 = call-dynamic "EnqueueMain.vi"("object in"=w486, "Message"="CoriolisMeasure") -> ("object out"=w485:refnum<class "Application.lvclass">)  [unwired: 16 in, 1 out]
      }
      event "Center ROI": Value Change {
        n183 = event-data() -> ()  [unwired: 1 in, 1 out]
        n184 = call-dynamic "EnqueueMain.vi"("object in"=w491, "Message"="HamamatsuCenterROI", "error in (no error)"=w487) -> ("object out"=w490:refnum<class "Application.lvclass">, "error out"=w488:errorcluster)  [unwired: 15 in]
      }
      event "StartLive": Value Change {
        n185 = event-data() -> ()  [unwired: 1 in, 1 out]
        n186 = call-dynamic "EnqueueMain.vi"("object in"=w496, "Message"="HamamatsuStartLive", "error in (no error)"=w492) -> ("object out"=w495:refnum<class "Application.lvclass">, "error out"=w493:errorcluster)  [unwired: 15 in]
      }
      event "Stop Live": Value Change {
        n187 = event-data() -> ()  [unwired: 1 in, 1 out]
        n188 = call-dynamic "EnqueueMain.vi"("object in"=w501, "Message"="HamamatsuStopLive", "error in (no error)"=w497) -> ("object out"=w500:refnum<class "Application.lvclass">, "error out"=w498:errorcluster)  [unwired: 15 in]
      }
      event "Configure ROI": Value Change {
        n189 = event-data() -> ()  [unwired: 1 in, 1 out]
        n190 = call-dynamic "EnqueueMain.vi"("object in"=w506, "Message"="HamamatsuConfigureROI", "error in (no error)"=w502) -> ("object out"=w505:refnum<class "Application.lvclass">, "error out"=w503:errorcluster)  [unwired: 15 in]
      }
      event "Read Redout Time": Value Change {
        n191 = event-data() -> ()  [unwired: 1 in, 1 out]
        n192 = call-dynamic "EnqueueMain.vi"("object in"=w511, "Message"="HamamatsuGetReadoutTime", "error in (no error)"=w507) -> ("object out"=w510:refnum<class "Application.lvclass">, "error out"=w508:errorcluster)  [unwired: 15 in]
      }
      event "Set Exposure Time": Value Change {
        n193 = event-data() -> ()  [unwired: 1 in, 1 out]
        n194 = call-dynamic "EnqueueMain.vi"("object in"=w516, "Message"="HamamatsuSetExposureTime", "error in (no error)"=w512) -> ("object out"=w515:refnum<class "Application.lvclass">, "error out"=w513:errorcluster)  [unwired: 15 in]
      }
      event "Open DIO signal helper": Value Change {
        n195 = event-data() -> ()  [unwired: 1 in, 1 out]
        n196 = Current VI's Path() -> (path=w523:path)
        n197 = Strip Path(path=w523) -> (stripped path=w526:path)  [unwired: 1 out]
        n198 = Build Path(base path=w526, name or relative path="VisualizeTriggerTiming.vi") -> (appended path=w524:path)
        n199 = Open VI Reference(type specifier VI Refnum (for type only)=refnum<vi> refnum, vi path=w524, options=128) -> (vi reference=w525:refnum<vi>)  [unwired: 3 in, 1 out]
        n200 = local read "Exposure (ms)"() -> (w530:dbl)
        n201 = local read "ReadoutTime"() -> (w531:dbl)
        n202 = invoke class="VI (strict)" method="FP.Open"(reference=w525, "Activate"=TRUE ("Activate?"), "State"=T16."Standard") -> (reference out=w527:refnum<vi>)  [unwired: 2 in, 4 out]
        n203 = local read "Triggering"() -> (w517:T9)
        n204 = call-by-ref "Start Asynchronous Call"(reference=w527, "Pulse Settings"=w517, "Exposure Time (ms)"=w530, "ReadoutTime"=w531) -> (reference out=w528:refnum<vi>, error out=w529:errorcluster)  [unwired: 17 in, 1 out]
        n205 = Close Reference(reference=w528, error in (no error)=w529) -> ()  [unwired: 1 out]
      }
      event "ReferenceMove": Value Change {
        n206 = event-data() -> ()  [unwired: 1 in, 1 out]
        n207 = call-dynamic "EnqueueMain.vi"("object in"=w538, "Message"="CetoniReferenceMove", "error in (no error)"=w534) -> ("object out"=w537:refnum<class "Application.lvclass">, "error out"=w535:errorcluster)  [unwired: 15 in]
      }
      event "ReadStatus": Value Change {
        n208 = event-data() -> ()  [unwired: 1 in, 1 out]
        n209 = call-dynamic "EnqueueMain.vi"("object in"=w543, "Message"="CetoniReadStatus", "error in (no error)"=w539) -> ("object out"=w542:refnum<class "Application.lvclass">, "error out"=w540:errorcluster)  [unwired: 15 in]
      }
      event "ConfigureSyringe": Value Change {
        n210 = event-data() -> ()  [unwired: 1 in, 1 out]
        n211 = call-dynamic "EnqueueMain.vi"("object in"=w549, "Message"="CetoniConfigureSyringe", "Message Data"="SyringeSettings", "error in (no error)"=w545) -> ("object out"=w548:refnum<class "Application.lvclass">, "error out"=w546:errorcluster)  [unwired: 14 in]
      }
      event "Stop ALL Pumps": Value Change {
        n212 = event-data() -> ()  [unwired: 1 in, 1 out]
        n213 = call-dynamic "EnqueueMain.vi"("object in"=w554, "Message"="CetoniStopAllSyringes", "error in (no error)"=w550) -> ("object out"=w553:refnum<class "Application.lvclass">, "error out"=w551:errorcluster)  [unwired: 15 in]
      }
      event "Syringe (only for syringe helper)": Value Change {
        n214 = event-data() -> ()  [unwired: 1 in, 2 out]
        n215 = call-dynamic "BDSyringeHelper.vi"("object in"=refnum<class "CetoniPump.lvclass"> refnum, "Syringe"="Syringe (only for syringe helper)") -> ("output cluster"=→"Syringe Helper":T6)  [unwired: 15 in, 2 out]
      }
      event "Go to Level": Value Change {
        n216 = event-data() -> ()  [unwired: 1 in, 1 out]
        n217 = call-dynamic "EnqueueMain.vi"("object in"=w564, "Message"="CetoniGoToLevel", "Message Data"="Go to Level", "error in (no error)"=w560) -> ("object out"=w563:refnum<class "Application.lvclass">, "error out"=w561:errorcluster)  [unwired: 14 in]
      }
      event "Inject Error<Replace Me>": Value Change {
        # "#CodeNeeded - Send the appropriate message for this user interface event."
        n218 = event-data() -> ()  [unwired: 1 in, 1 out]
        n219 = call-dynamic "EnqueueMain.vi"("object in"=w570, "Message"="InjectError", "Message Data"=errorcluster {"status"=TRUE, "code"=-8000, "source"="Injected Error"} ("error in (no error)"), "error in (no error)"=w566) -> ("object out"=w569:refnum<class "Application.lvclass">, "error out"=w567:errorcluster)  [unwired: 14 in]
      }
      event Panel Close? {
        # "Send the 'Confirm Quit' message if the user closes the panel of the VI. Discard the event so the 'Confirm Quit' message has a chance to run."
        n220 = event-data() -> ()  [unwired: 1 in, 1 out]
        n221 = call-dynamic "EnqueueMain.vi"("object in"=w572, "Message"="Confirm Quit", "error in (no error)"=w574, "Priority Message? (F)"=TRUE) -> ("object out"=w571:refnum<class "Application.lvclass">, "error out"=w573:errorcluster)  [unwired: 14 in]
        n222 = event-data("Discard?"=TRUE) -> ()  [unwired: 1 in, 1 out]
      }
      event Application Instance Close {
        # "#CodeRecommended - When a project closes, all VIs within that project are aborted and leave memory. However, any code placed in this event frame is guaranteed to run to completion, so add any cleanup code that absolutely must happen here."
        n223 = event-data() -> ()  [unwired: 1 in, 1 out]
      }
      event "Exit": Value Change {
        n224 = event-data() -> ()  [unwired: 1 in, 1 out]
        n225 = call-dynamic "EnqueueMain.vi"("object in"=w585, "Message"="Exit", "error in (no error)"=w581, "Priority Message? (F)"=TRUE) -> ("object out"=w584:refnum<class "Application.lvclass">, "error out"=w580:errorcluster)  [unwired: 14 in]
      }
      event User Event {
        (unwired) "\"Exit\" button pressed" ("VI Stopped")
        # "The Message Handling Loop processed an \"Exit\" message, which fired this event to stop the Event Handling Loop."
        n226 = event-data() -> ()  [unwired: 1 in, 1 out]
      }
      event User Event {
        n227 = event-data() -> ("Message"=w591:string, "Message Data"=w588:variant)  [unwired: 1 in]
        n228 = case shown="Default" w591 {
          tunnel: w590 -> [w596 w597 w604 w622]
          tunnel: [w596 w597 w600 w619] -> w589
          tunnel: w588 -> [w595 _ w606 w623]
          frame "UpdateStatus" {
            n229 = Variant To Data(type="" ("Status"), Variant=w595) -> (data=→"Status":string)  [unwired: 1 in, 1 out]
          }
          frame Default {
          }
          frame "UpdateLive" {
            w599 = 0 ("Window Number (0...15)")
            n230 = Variant To Data(error in=w604, type=T15 refnum ("FreeRunningImage"), Variant=w606) -> (data=w603:T15, error out=w602:errorcluster)
            n231 = call "IMAQ WindShow"("error in (no error)"=w602, "Get/Set Status? (Set)"=FALSE, "Window Number (0...15)"=w599) -> ("error out"=w601:errorcluster, "Visible?"=w598:bool)  [unwired: 3 in, 1 out]
            n232 = case shown="True" w598 {
              tunnel: w603 -> [_ w612]
              tunnel: w601 -> [w608 w611]
              tunnel: [w608 w610] -> w600
              tunnel: w599 -> [_ w609]
              frame False {
              }
              frame True {
                n233 = call "IMAQ WindDraw"("Resize to Image Size? (Y)"=FALSE, "Window Number (0...15)"=w609, "error in (no error)"=w611, "Title"="Live Image", "Image"=w612) -> ("error out"=w610:errorcluster)  [unwired: 5 in, 1 out]
              }
            }
          }
          frame "UpdateHWTimed" {
            n234 = Variant To Data(error in=w622, type=T15[] [] ("HWSyncedImages"), Variant=w623) -> (data=w621:T15[], error out=w620:errorcluster)
            n235 = Build Array("Frame1" ("Title"), "Frame2" ("Title")) -> (w615:string[])
            n236 = for {
              tunnel: w621 -> [w631] mode=indexing
              shift-right: [w628] -> w619
              shift-left: w620 -> [w630]
              tunnel: w615 -> [w624] mode=indexing
              i -> [w626]
              n237 = Increment(x=w626) -> (x+1=w625:i32)
              n238 = call "IMAQ WindShow"("error in (no error)"=w630, "Get/Set Status? (Set)"=FALSE, "Window Number (0...15)"=w625) -> ("error out"=w629:errorcluster, "Visible?"=w627:bool)  [unwired: 3 in, 1 out]
              n239 = case shown="True" w627 {
                tunnel: w631 -> [_ w638]
                tunnel: w629 -> [w633 w637]
                tunnel: [w633 w636] -> w628
                tunnel: w625 -> [_ w635]
                tunnel: w624 -> [_ w634]
                frame False {
                }
                frame True {
                  n240 = call "IMAQ WindDraw"("Resize to Image Size? (Y)"=FALSE, "Window Number (0...15)"=w635, "error in (no error)"=w637, "Title"=w634, "Image"=w638) -> ("error out"=w636:errorcluster)  [unwired: 5 in, 1 out]
                }
              }
            }
          }
        }
      }
    }
    n241 = call-dynamic "ErrorHandlerEventLoop.vi"("object in"=w459, "error in (no error)"=w461) -> ("object out"=w458:refnum<class "Application.lvclass">, "error out"=w460:errorcluster)  [unwired: 16 in]
  }
  n242 = disable-structure shown="Disabled" {
    frame Disabled {
      n243 = call "VisualizeTriggerTiming.vi"() -> ()  [unwired: 19 in, 1 out]
    }
    frame Enabled {
    }
  }
  n244 = Merge Errors(w7, w8) -> (w6:errorcluster)
  n245 = call-dynamic "CleanUp.vi"("object in"=w9, "error in (no error)"=w6) -> ("error out"=→"error out":errorcluster)  [unwired: 16 in, 1 out]
